vi "显示一组测试数据-输入为Cluster.vi"(6 "量测项名称":string[](array[string]), 7 "Font, Size & Style":T1={"Desired Font (Application)"=enum."User-specified Font", "[User-specified Font]"={"Font Name"="", "Size"=120, "Strikeout?"=FALSE, "Italic?"=FALSE, "Underline?"=FALSE, "Outline?"=FALSE, "Shadow?"=FALSE, "Bold?"=FALSE, "Rotation Angle"=0.0}, "Horizontal Alignment"=0, "Vertical Alignment"=0} {"Horizontal Alignment" items=["Left", "Center", "Right"]; "Vertical Alignment" items=["Bottom", "Top", "Baseline"]}, 8 "显示坐标":cluster{dbl, "Numeric":dbl}[](array[cluster])=[{300.0, "Numeric"=200.0}, {300.0, "Numeric"=400.0}, {300.0, "Numeric"=600.0}, {300.0, "Numeric"=800.0}, {300.0, "Numeric"=1000.0}, {300.0, "Numeric"=1200.0}, {300.0, "Numeric"=1400.0}], 10 "存档数据":T3, 11 "Img":T2) -> (3 "Img out":T2 caption="Imgout")   [LabVIEW 2014]
uses:
  <vilib>/vision/Image Controls.llb/IMAQ Image.ctl
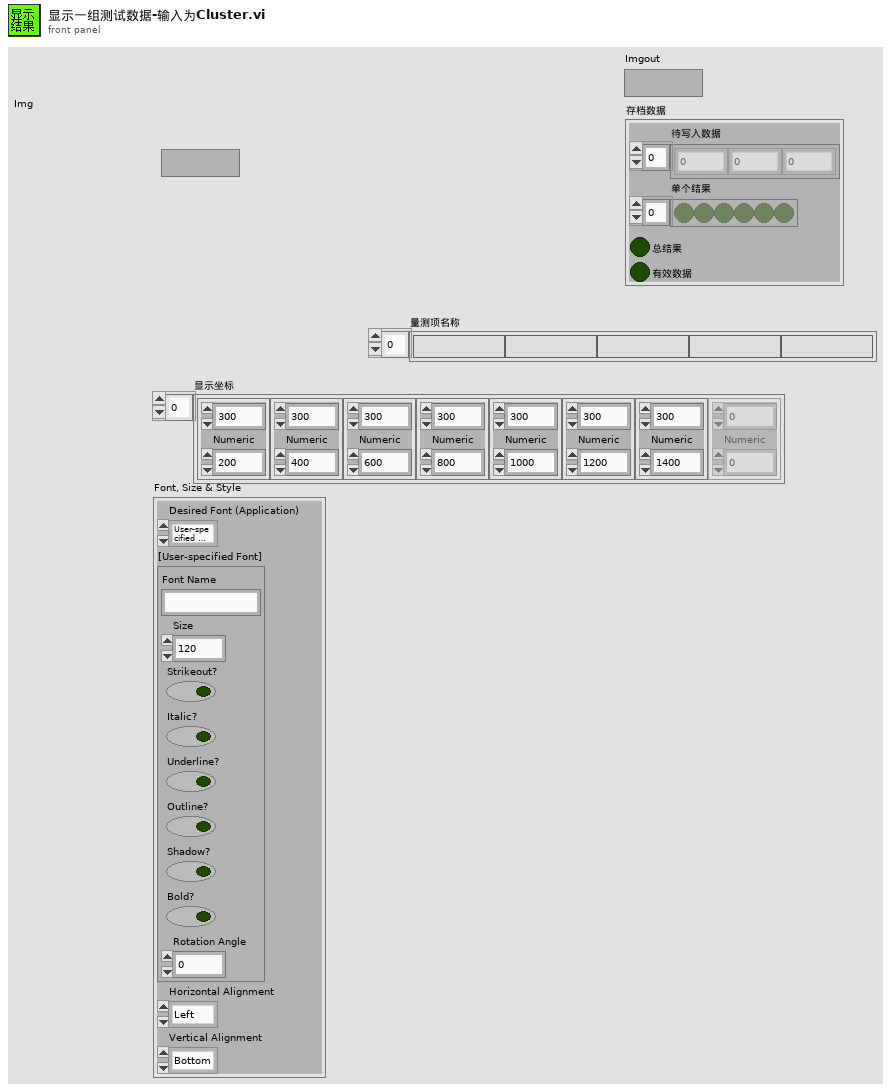
[diagram p1: front panel]
types:
  T1 = cluster{"Desired Font (Application)":enum16{"User-specified Font", "Application Font", "System Font", "Dialog Font"}, "[User-specified Font]":cluster{"Font Name":string, "Size":i16, "Strikeout?":bool, "Italic?":bool, "Underline?":bool, "Outline?":bool, "Shadow?":bool, "Bold?":bool, "Rotation Angle":dbl}, "Horizontal Alignment":i16, "Vertical Alignment":i16}
  T2 = typedef "IMAQ Image.ctl" = refnum<image>
  T3 = typedef "控件-存档数据和结果.ctl" = cluster{"待写入数据":dbl[], "单个结果":bool[], "总结果":bool, "有效数据":bool}
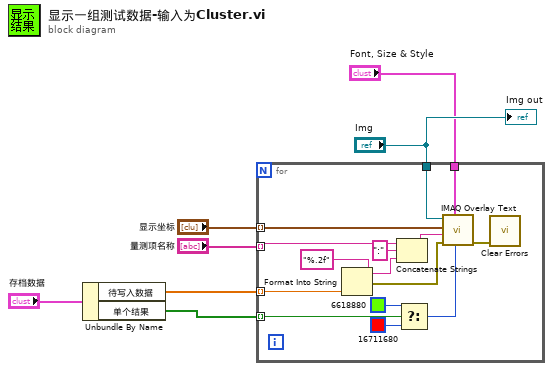
[diagram p0: block diagram]
diagram:
  n1 = Unbundle By Name("存档数据") -> ("待写入数据"=w2:dbl[], "单个结果"=w1:bool[])
  n2 = for {
    tunnel: "Img" -> [w22]
    tunnel: w2 -> [w21] mode=indexing
    tunnel: "显示坐标" -> [w19] mode=indexing
    tunnel: w1 -> [w20] mode=indexing
    tunnel: "Font, Size & Style" -> [w18]
    tunnel: "量测项名称" -> [w17] mode=indexing
    n3 = Format Into String(format string="%.2f" ("格式字符串"), w21) -> (resulting string=w9:string, error out=w12:errorcluster)  [unwired: 2 in]
    n4 = Concatenate Strings(w17, ":" ("字符串"), w9) -> (w10:string)
    n5 = Select(t=u32 6618880 ("Text Color (black)"), s=w20, f=u32 16711680 ("Text Color (black)")) -> (s? t:f=w13:u32)
    n6 = call "IMAQ Overlay Text"("Text Color (black)"=w13, "Font, Size & Style"=w18, "error in (no error)"=w12, "String"=w10, "Origin"=w19, "Image"=w22) -> ("error out"=w11:errorcluster)  [unwired: 4 in, 1 out]
    n7 = call <vilib>:"Clear Errors.vi"("error in (no error)"=w11) -> ()  [unwired: 5 in, 2 out]
  }
  "Img out" <- "Img"
